vi "parse and check websocket headers.vi"(7 "accept key":string, 8 "error in":errorcluster, 9 "timeout ms":i32, 10 "max header size":i32, 11 "TCP Network Connection in":refnum<k5>) -> (0 "error out":errorcluster, 3 "headers":T1)   [LabVIEW 2016, in "websocket client.lvclass"]
uses:
  websocket client.lvclass
  HTTP headers/http header data.ctl
  HTTP headers/http headers.lvlib
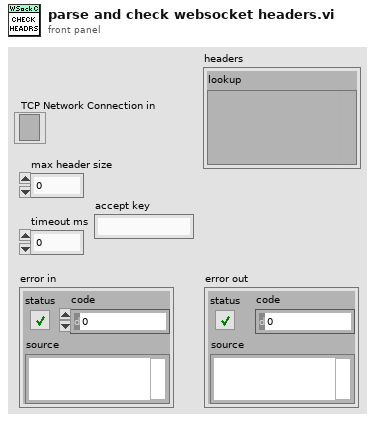
[diagram p1: front panel]
types:
  T1 = typedef "http headers.lvlib/http header data.ctl" = cluster{"lookup":variant}
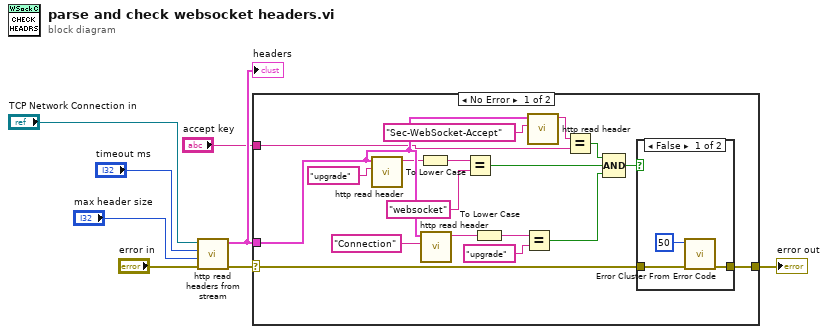
[diagram p0: block diagram]
diagram:
  n1 = call "http read headers from stream.vi"("error in"="error in", "max header size"="max header size", "timeout ms"="timeout ms", "TCP Network Connection in"="TCP Network Connection in") -> ("error out"=w6:errorcluster, "headers"=w8:T1)  [unwired: 6 in]
  "headers" <- w8
  n2 = case shown="No Error" w6 {
    selector: w6 -> [w11 w31]
    tunnel: w8 -> [w26 _]
    tunnel: [w12 w31] -> w7
    tunnel: "accept key" -> [w10 _]
    frame No Error {
      n3 = call "http read header.vi"("header field name"="upgrade", "headers"=w26) -> ("value"=w23:string)  [unwired: 8 in, 1 out]
      n4 = To Lower Case(string=w23) -> (all lower case string=w9:string)
      n5 = call "http read header.vi"("header field name"="Connection", "headers"=w26) -> ("value"=w17:string)  [unwired: 8 in, 1 out]
      n6 = Equal?(x=w9, y="websocket") -> (x = y?=w19:bool)
      n7 = To Lower Case(string=w17) -> (all lower case string=w16:string)
      n8 = Equal?(x=w16, y="upgrade") -> (x = y?=w14:bool)
      n9 = call "http read header.vi"("header field name"="Sec-WebSocket-Accept", "headers"=w26) -> ("value"=w24:string)  [unwired: 8 in, 1 out]
      n10 = Equal?(x=w24, y=w10) -> (x = y?=w20:bool)
      n11 = Compound Arithmetic op=AND(w20, w19, w14) -> (w13:bool)
      n12 = case shown="False" w13 {
        tunnel: [w28 w30] -> w12
        tunnel: w11 -> [w29 w30]
        frame False {
          n13 = call <vilib>:"Error Cluster From Error Code.vi"("error in (no error)"=w29, "error code (0)"=50) -> ("error out"=w28:errorcluster)  [unwired: 7 in]
        }
        frame True {
        }
      }
    }
    frame Error {
    }
  }
  "error out" <- w7
